vi "Configure Arbitrary Waveform.vi"(6 "Sample Rate (16.384 MSa/s)":dbl=16384000.0, 7 "Interpolation (Zero-Order Hold)":u16(ring) items=["Zero-Order Hold", "Linear"], 8 "error in (no error)":errorcluster, 9 "Arb Mode (TrueArb)":u16(ring) items=["TrueArb", "DDS"], 10 "Channel (1:Channel 1)":i32(ring)=1 items=["Channel 1"=1, "Channel 2"=2], 11 "VISA resource name":refnum<visa-resource-name>) -> (0 "error out":errorcluster, 3 "VISA resource name out":refnum<visa-resource-name>)   [LabVIEW 2015, in "Siglent SDG X Series.lvlib"]
doc: "Sets the waveform parameters for an arbitrary waveform."
uses:
  <instrlib>/Siglent SDG X Series/Siglent SDG X Series.lvlib
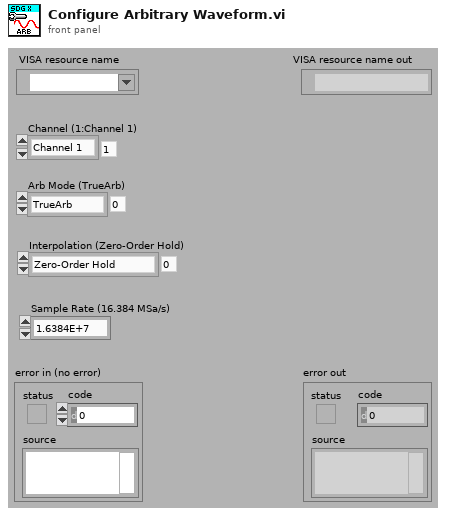
[diagram p1: front panel]
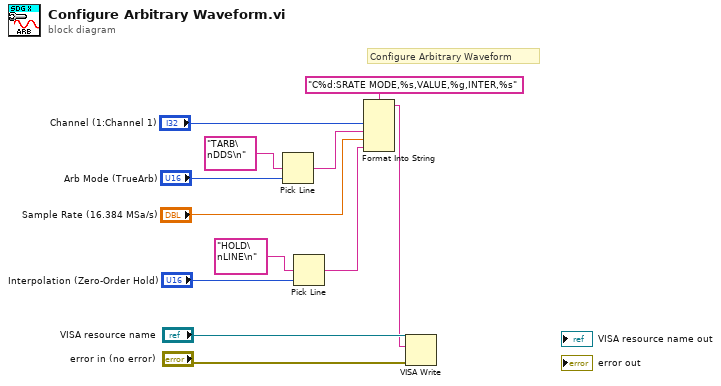
[diagram p0: block diagram]
diagram:
  # "Configure Arbitrary Waveform"
  n1 = Pick Line(multi-line string="TARB\nDDS\n" ("多行字符串"), line index="Arb Mode (TrueArb)") -> (output string=w4:string)  [unwired: 1 in]
  n2 = Pick Line(multi-line string="HOLD\nLINE\n" ("多行字符串"), line index="Interpolation (Zero-Order Hold)") -> (output string=w1:string)  [unwired: 1 in]
  n3 = Format Into String(format string="C%d:SRATE MODE,%s,VALUE,%g,INTER,%s", "Channel (1:Channel 1)", w4, "Sample Rate (16.384 MSa/s)", w1) -> (resulting string=w9:string)  [unwired: 2 in, 1 out]
  n4 = VISA Write(VISA resource name="VISA resource name", write buffer=w9, error in (no error)="error in (no error)") -> ()  [unwired: 3 out]
